vi "Control Down.vi"(8 "error in (no error)":errorcluster) -> (0 "error out":errorcluster)   [LabVIEW 2015, in "LVJSON.lvlib" / "Shared.lvlib"]
uses:
  Shared.lvlib
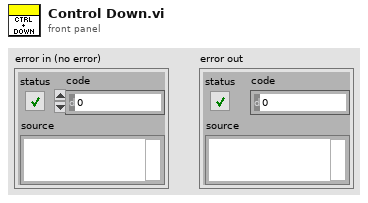
[diagram p1: front panel]
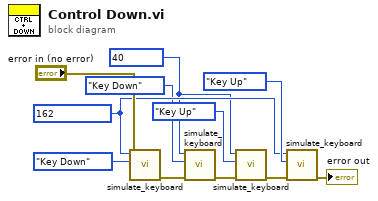
[diagram p0: block diagram]
diagram:
  w4 = u8 40 ("Virtual Key")
  w8 = u8 162 ("Virtual Key")
  n1 = call "simulate_keyboard.vi"("error in (no error)"="error in (no error)", "Direction"=enum16{"Key Down", "Key Up"}."Key Down", "Virtual Key"=w8) -> ("error out"=w1:errorcluster)  [unwired: 7 in]
  n2 = call "simulate_keyboard.vi"("error in (no error)"=w1, "Direction"=enum16{"Key Down", "Key Up"}."Key Down", "Virtual Key"=w4) -> ("error out"=w3:errorcluster)  [unwired: 7 in]
  n3 = call "simulate_keyboard.vi"("error in (no error)"=w3, "Direction"=enum16{"Key Down", "Key Up"}."Key Up", "Virtual Key"=w4) -> ("error out"=w7:errorcluster)  [unwired: 7 in]
  n4 = call "simulate_keyboard.vi"("error in (no error)"=w7, "Direction"=enum16{"Key Down", "Key Up"}."Key Up", "Virtual Key"=w8) -> ("error out"=→"error out":errorcluster)  [unwired: 7 in]
